vi "Determine Warnings - Copy(3-5).vi"(8 "error in (no error)":errorcluster, 9 "Min Temp":dbl, 10 "Max Temp":dbl, 11 "Current Temp":dbl) -> (0 "error out":errorcluster, 1 "Warning?":bool, 2 "Warning Text":string)   [LabVIEW 2015]
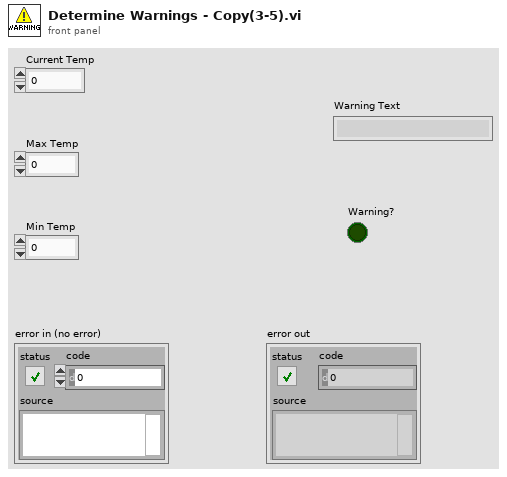
[diagram p1: front panel]
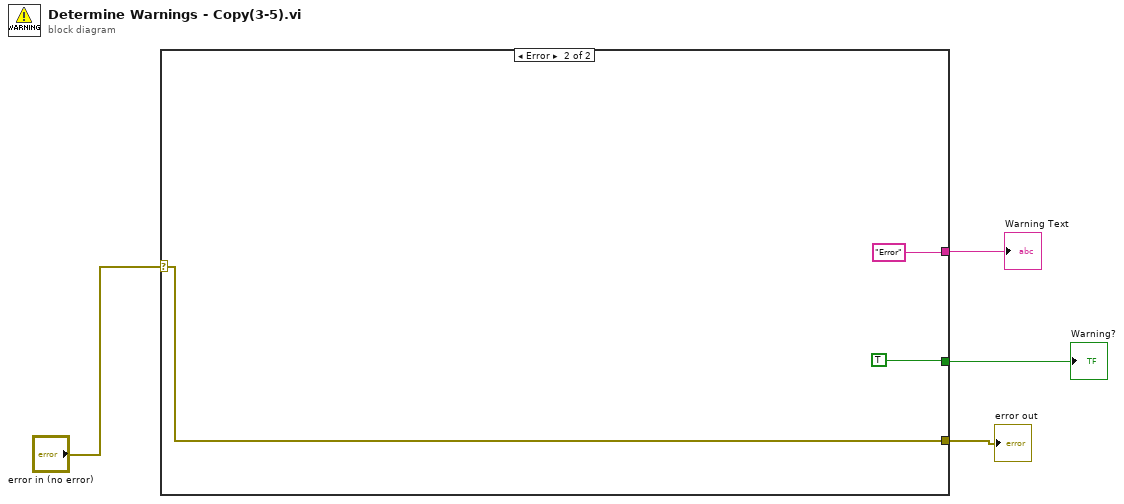
[diagram p0: block diagram]
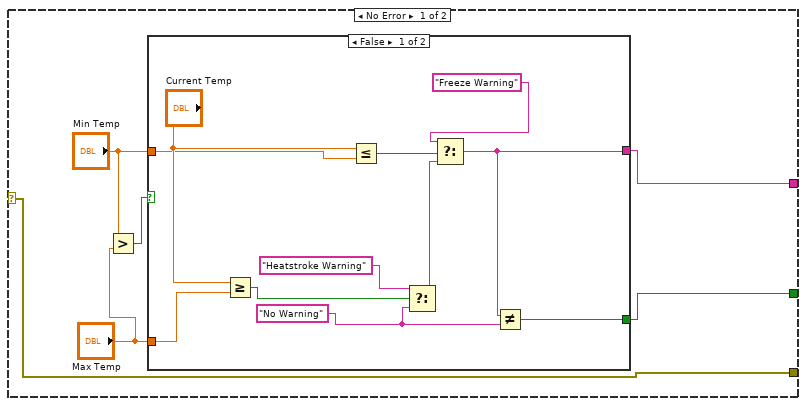
[diagram p2: hidden frame]
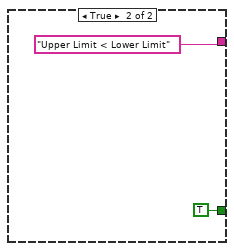
[diagram p3: hidden frame]
diagram:
  n1 = case shown="Error" "error in (no error)" {
    selector: "error in (no error)" -> [w5 w24]
    tunnel: [w7 "Error"] -> w4
    tunnel: [w6 TRUE] -> w3
    tunnel: [w5 w24] -> w2
    frame No Error {
      n2 = Greater?(x="Min Temp", y="Max Temp") -> (0:w8:bool)
      n3 = case shown="False" w8 {
        tunnel: [w18 TRUE] -> w6
        tunnel: [w14 "Upper Limit < Lower Limit"] -> w7
        tunnel: "Min Temp" -> [w12 _]
        tunnel: "Max Temp" -> [w11 _]
        frame False {
          w20 = "No Warning"
          n4 = Greater Or Equal?(x="Current Temp", y=w11) -> (x >= y?=w13:bool)
          n5 = Less Or Equal?(x="Current Temp", y=w12) -> (x <= y?=w15:bool)
          n6 = Select(t="Heatstroke Warning", s=w13, f=w20) -> (s? t:f=w16:string)
          n7 = Select(t="Freeze Warning", s=w15, f=w16) -> (s? t:f=w14:string)
          n8 = Not Equal?(x=w14, y=w20) -> (x != y?=w18:bool)
        }
        frame True {
        }
      }
    }
    frame Error {
    }
  }
  "Warning?" <- w3
  "Warning Text" <- w4
  "error out" <- w2
